vi "ANA_Pin_config.vi"(11 "Pin_Config":i32) -> (0 "Boolean":bool, 1 "ADC_Channel":u16[](array[numeric]), 3 "ADC":T1[](array[typedef]), 4 "ADC+CH":string[](array[string]))   [LabVIEW 2019]
uses:
  ADC/Labview/Ctrls/ADC_CTRL.ctl
panel:
  out "ADC 2":T1
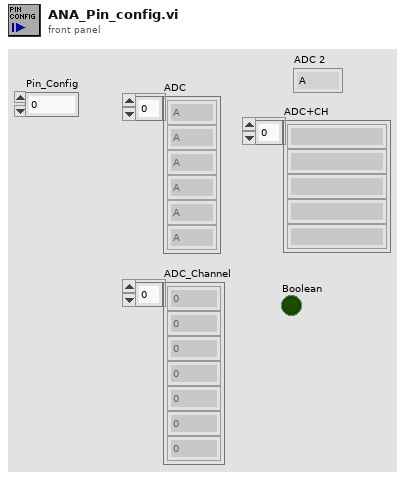
[diagram p1: front panel]
types:
  T1 = typedef "ADC_CTRL.ctl" = enum16{"A", "B", "C"}
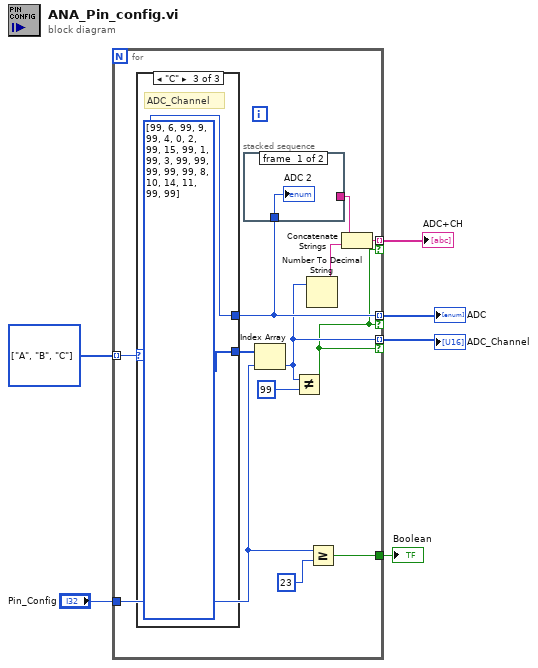
[diagram p0: block diagram]
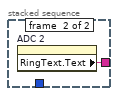
[diagram p2: hidden frame]
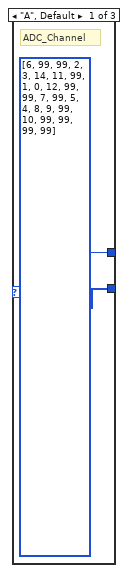
[diagram p3: hidden frame]
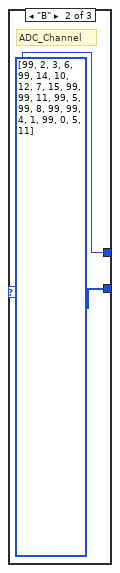
[diagram p4: hidden frame]
diagram:
  w6 = T1[] [enum."A", enum."B", enum."C"] items=["A", "B", "C"]
  n1 = for {
    tunnel: w6 -> [w18] mode=indexing
    tunnel: "Pin_Config" -> [w9]
    tunnel: [w14] -> w3 mode=indexing if=w10
    tunnel: [w15] -> w4 mode=indexing if=w10
    tunnel: [w11] -> w2 mode=indexing if=w10
    tunnel: [w7] -> w1
    n2 = case shown="\"C\"" w18 {
      selector: w18 -> [w21 w23 w25]
      tunnel: [u16[] [6, 99, 99, 2, 3, 14, 11, 99, 1, 0, 12, 99, 99, 7, 99, 5, 4, 8, 9, 99, 10, 99, 99, 99, 99] u16[] [99, 2, 3, 6, 99, 14, 10, 12, 7, 15, 99, 99, 11, 99, 5, 99, 8, 99, 99, 4, 1, 99, 0, 5, 11] u16[] [99, 6, 99, 9, 99, 4, 0, 2, 99, 15, 99, 1, 99, 3, 99, 99, 99, 99, 99, 8, 10, 14, 11, 99, 99]] -> w16
      tunnel: [w21 w23 w25] -> w15
      frame "A", Default {
        # "ADC_Channel"
      }
      frame "B" {
        # "ADC_Channel"
      }
      frame "C" {
        # "ADC_Channel"
      }
    }
    n3 = stacked-sequence {
      tunnel: w15 -> [w19 _]
      tunnel: [_ w20] -> w13
      frame #0 {
        "ADC 2" <- w19
      }
      frame #1 {
        n4 = property on="ADC 2" class="Enum (strict)"() -> ("RingText.Text"=w20:string)  [unwired: 2 in, 2 out]
      }
    }
    n5 = Index Array(array=w16, index=w9) -> (element=w14:u16)
    n6 = Not Equal?(x=w14, y=99) -> (x != y?=w10:bool)
    n7 = Number To Decimal String(number=w14) -> (decimal integer string=w12:string)  [unwired: 1 in]
    n8 = Greater Or Equal?(x=w9, y=23) -> (x >= y?=w7:bool)
    n9 = Concatenate Strings(w13, w12) -> (w11:string)
  }
  "ADC" <- w4
  "ADC_Channel" <- w3
  "ADC+CH" <- w2
  "Boolean" <- w1
